vi "sub_file_log_2.vi"(0 "LOG PATH IN":path, 1 "TIMESTAMP":timestamp format="%<%x %.3X>T", 2 "UID":string, 3 "ACTIVITY":string) -> (14 "LOG PATH OUT":path, 19 "ERROR OUT":errorcluster)   [LabVIEW 2018]
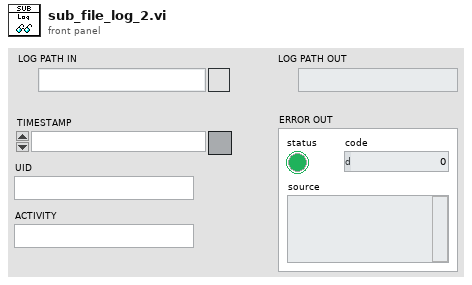
[diagram p1: front panel]
types:
  T1 = enum16{"open", "replace", "create", "open or create", "replace or create", "replace or create with confirmation"}
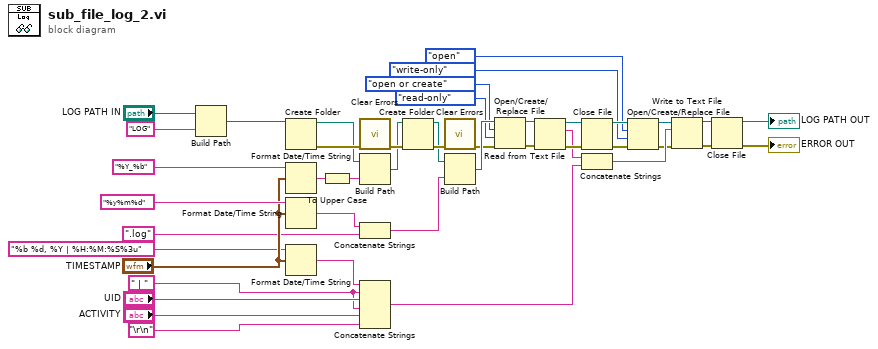
[diagram p0: block diagram]
diagram:
  w33 = " | " ("string")
  n1 = Build Path(base path="LOG PATH IN", name or relative path="LOG" ("string")) -> (appended path=w42:path)
  n2 = Create Folder(path (use dialog)=w42) -> (created path=w28:path, error out=w30:errorcluster)  [unwired: 2 in, 1 out]
  n3 = Format Date/Time String(time format string (%c)="%Y_%b", seconds (now)="TIMESTAMP") -> (date/time string=w19:string)  [unwired: 1 in]
  n4 = Format Date/Time String(time format string (%c)="%y%m%d", seconds (now)="TIMESTAMP") -> (date/time string=w21:string)  [unwired: 1 in]
  n5 = Format Date/Time String(time format string (%c)="%b %d, %Y | %H:%M:%S%3u", seconds (now)="TIMESTAMP") -> (date/time string=w1:string)  [unwired: 1 in]
  n6 = To Upper Case(1:w19) -> (0:w20:string)
  n7 = call <vilib>:"Clear Errors.vi"("error in (no error)"=w30) -> ("error out"=w29:errorcluster)  [unwired: 5 in, 1 out]
  n8 = Build Path(base path=w28, name or relative path=w20) -> (appended path=w27:path)
  n9 = Concatenate Strings(w21, ".log" ("string")) -> (w24:string)
  n10 = Concatenate Strings(w1, w33, "UID", w33, "ACTIVITY", "\r\n") -> (w2:string)
  n11 = Create Folder(path (use dialog)=w27, error in=w29) -> (created path=w25:path, error out=w26:errorcluster)  [unwired: 1 in, 1 out]
  n12 = call <vilib>:"Clear Errors.vi"("error in (no error)"=w26) -> ("error out"=w22:errorcluster)  [unwired: 5 in, 1 out]
  n13 = Build Path(base path=w25, name or relative path=w24) -> (appended path=w23:path)
  n14 = Open/Create/Replace File(file path (use dialog)=w23, error in=w22, operation (0:open)=T1."open or create", access (0:read/write)=enum16{"read/write", "read-only", "write-only"}."read-only") -> (refnum out=w15:refnum<file>, error out=w16:errorcluster)  [unwired: 2 in, 1 out]
  n15 = Read from Text File(file (use dialog)=w15, error in=w16) -> (refnum out=w13:refnum<file>, text=w12:string, error out=w14:errorcluster)  [unwired: 2 in, 1 out]
  n16 = Close File(refnum=w13, error in=w14) -> (path=w10:path, error out=w11:errorcluster)
  n17 = Concatenate Strings(w12, w2) -> (w9:string)
  n18 = Open/Create/Replace File(file path (use dialog)=w10, error in=w11, operation (0:open)=T1."open", access (0:read/write)=enum16{"read/write", "read-only", "write-only"}."write-only") -> (refnum out=w7:refnum<file>, error out=w8:errorcluster)  [unwired: 2 in, 1 out]
  n19 = Write to Text File(file (use dialog)=w7, text=w9, error in=w8) -> (refnum out=w17:refnum<file>, error out=w18:errorcluster)  [unwired: 1 in, 1 out]
  n20 = Close File(refnum=w17, error in=w18) -> (path=→"LOG PATH OUT":path, error out=→"ERROR OUT":errorcluster)
